vi "Is Empty Array.vi"(1 "Deserialized JSON Data":variant) -> (0 "Empty Array?":bool)   [LabVIEW 2020, in "JKI JSON Serialization.lvlib"]
uses:
  JKI JSON Serialization.lvlib
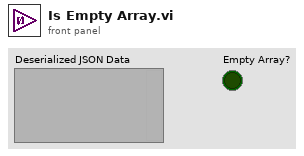
[diagram p1: front panel]
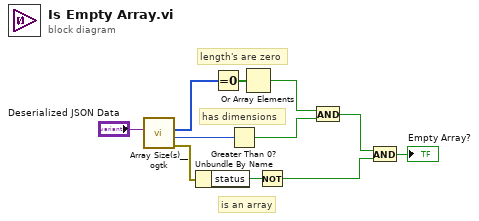
[diagram p0: block diagram]
diagram:
  # "has dimensions"
  # "length's are zero"
  # "is an array"
  n1 = call <userlib>:"Array Size(s)__ogtk.vi"("Array"="Deserialized JSON Data") -> ("error out"=w10:errorcluster, "N dims"=w3:u32, "Size(s)"=w9:u32[])  [unwired: 8 in]
  n2 = Unbundle By Name(w10) -> ("status"=w7:bool)
  n3 = Equal To 0?(x=w9) -> (x = 0?=w8:bool[])
  n4 = Greater Than 0?(x=w3) -> (x > 0?=w2:bool)
  n5 = Or Array Elements(Boolean array=w8) -> (logical OR=w1:bool)
  n6 = Not(x=w7) -> (.not. x?=w6:bool)
  n7 = And(x=w1, y=w2) -> (x .and. y?=w4:bool)
  n8 = And(x=w4, y=w6) -> (x .and. y?=→"Empty Array?":bool)
